vi "Autonomous Independent.vi"   [LabVIEW 2016]
doc: "This VI is called when autonomous begins, and will automatically be terminated when autonomous ends. You can carry out timed or sensor driven robot movement independently without needing to return to the caller."
uses:
  <vilib>/Rock Robotics/WPI/Relay/WPI_RelayValue.ctl
  <vilib>/Rock Robotics/WPI/Utilities/WPI_GetSetVariantRefNum.vi
  <vilib>/Rock Robotics/Network Tables/NT Read String.vi
  <vilib>/Rock Robotics/Network Tables/NT Read Number.vi
  <vilib>/Rock Robotics/Network Tables/NT Write Numeric Array.vi
panel:
  # "Be sure to right-click and choose Data Operations>>Make Current Value default if you want to save the array values with the VI"
types:
  T1 = typedef "WPI_JoystickDevRef.ctl" = cluster{"Device":T2}
  T2 = typedef "WPI_JoystickDeviceEnum.ctl" = enum16{"USB 0", "USB 1", "USB 2", "USB 3", "USB 4", "USB 5"}
  T3 = typedef "WPI_ServoDeviceRef.ctl" = cluster{"DeviceStatus":errorcluster, "PWM Channel":T4, "DeadBand":T5}
  T4 = typedef "FPGA_DIOPWMChannel.ctl" = enum8{"PWM 0", "PWM 1", "PWM 2", "PWM 3", "PWM 4", "PWM 5", "PWM 6", "PWM 7", "PWM 8", "PWM 9", "PWM MXP 0", "PWM MXP 1", "PWM MXP 2", "PWM MXP 3", "PWM MXP 4", "PWM MXP 5", "PWM MXP 6", "PWM MXP 7", "PWM MXP 8", "PWM MXP 9", "Invalid"}
  T5 = typedef "WPI_PWMDeadband.ctl" = cluster{"Name":string, "maxPositivePwm":i32, "minPositivePwm":i32, "centerPwm":i32, "maxNegativePwm":i32, "minNegativePwm":i32, "angularRange":u16}
  T6 = typedef "WPI_RelayValue.ctl" = enum16{"Off", "On", "Forward", "Reverse"}
  T7 = typedef "WPI_SwitchDevRef.ctl" = cluster{"DevStatus":errorcluster, "DIO Channel":T8, "CntIndex":T9, "Normally Closed":bool}
  T8 = typedef "FPGA_DIOChannel.ctl" = enum8{"DIO 0", "DIO 1", "DIO 2", "DIO 3", "DIO 4", "DIO 5", "DIO 6", "DIO 7", "DIO 8", "DIO 9", "DIO MXP 0", "DIO MXP 1", "DIO MXP 2", "DIO MXP 3", "DIO MXP 4", "DIO MXP 5", "DIO MXP 6", "DIO MXP 7", "DIO MXP 8", "DIO MXP 9", "DIO MXP 10", "DIO MXP 11", "DIO MXP 12", "DIO MXP 13", "DIO MXP 14", "DIO MXP 15", "SPI Port CS1", "SPI Port CS2", "SPI Port CS3", "SPI Port MISO", "SPI Port MOSI", "Invalid"}
  T9 = typedef "FPGA_CounterCtrSystemIndex.ctl" = enum8{"Ctr 0", "Ctr 1", "Ctr 2", "Ctr 3", "Ctr 4", "Ctr 5", "Ctr 6", "Ctr 7", "Invalid"}
  T10 = typedef "WPI_RelayDevRef.ctl" = cluster{"DevStatus":errorcluster, "Relay Channel":T11, "Relay Direction":T12}
  T11 = typedef "FPGA_DIORelayChannel.ctl" = enum8{"Relay 0", "Relay 1", "Relay 2", "Relay 3", "Invalid"}
  T12 = typedef "WPI_RelayDirection.ctl" = enum16{"Both directions", "Forward only", "Reverse only"}
  T13 = typedef "WPI_RobotDriveDevRef.ctl" = cluster{"DevStatus":errorcluster, "Motors[]":T14[], "Square Inputs":bool, "Max Output":dbl}
  T14 = typedef "WPI_MotorControlDeviceRef.ctl" = cluster{"DeviceStatus":errorcluster, "Type":T15, "PWM":cluster{"PWM Channel":T4, "DeadBand":T5}, "CAN":cluster{"Device Number":u8, "SetOutput VI Ref":variant, "GetOutput VI Ref":variant, "Enable VI Ref":variant, "Disable VI Ref":variant, "Data":variant}, "Invert":bool}
  T15 = typedef "WPI_MotorControlType.ctl" = enum16{"PWM", "CAN"}
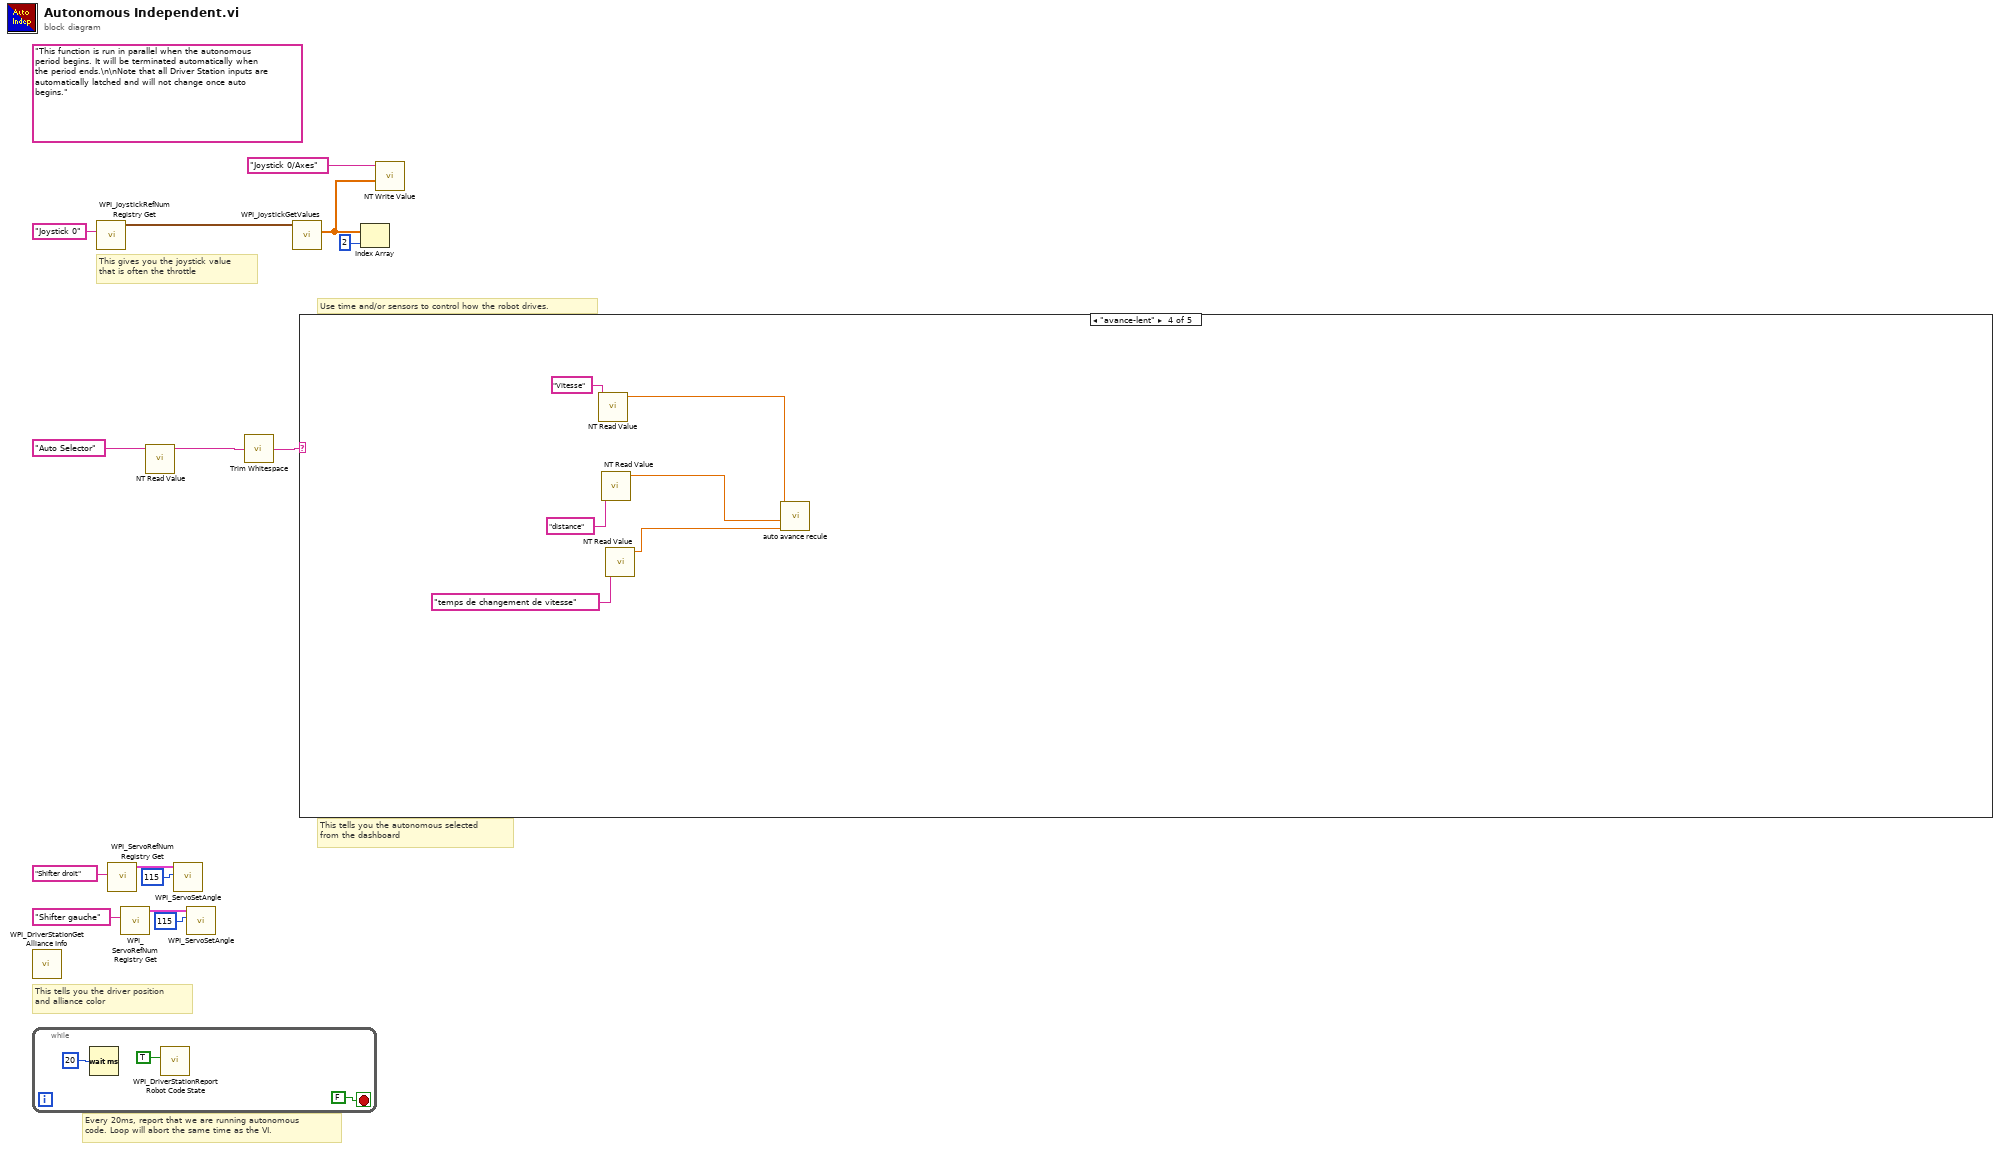
[diagram p0: block diagram]
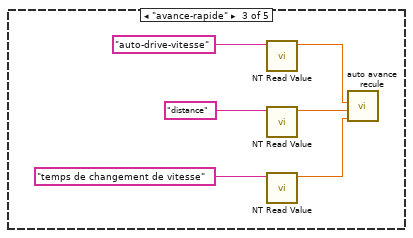
[diagram p4: hidden frame]
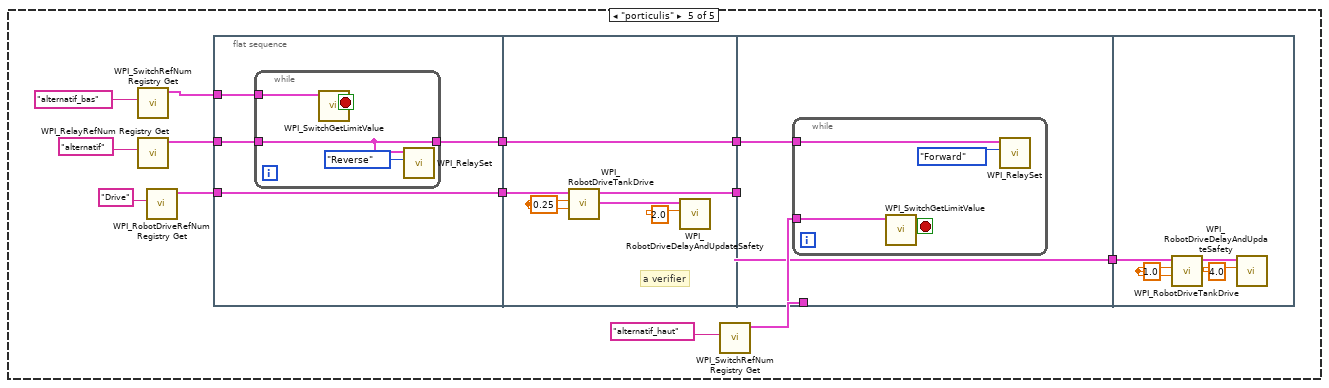
[diagram p5: hidden frame]
diagram:
  (unwired) "This function is run in parallel when the autonomous period begins. It will be terminated automatically when the period ends.\n\nNote that all Driver Station inputs are automatically latched and will not change once auto begins."
  # "This tells you the autonomous selected\nfrom the dashboard"
  # "Every 20ms, report that we are running autonomous\ncode. Loop will abort the same time as the VI."
  # "This gives you the joystick value\nthat is often the throttle"
  # "Use time and/or sensors to control how the robot drives."
  # "This tells you the driver position\nand alliance color"
  n1 = call <vilib>:"WPI_DriverStationGet Alliance Info.vi"() -> ()  [unwired: 12 out]
  n2 = while {
    stop <- FALSE stop-if-true
    n3 = Wait (ms)(milliseconds to wait=u32 20) -> ()  [unwired: 1 out]
    n4 = call <vilib>:"WPI_DriverStationReport Robot Code State.vi"("Autonomous"=TRUE) -> ()  [unwired: 10 in, 1 out]
  }
  n5 = call <vilib>:"WPI_JoystickRefNum Registry Get.vi"("refnum name"="Joystick 0") -> ("JoystickDevRef"=w13:T1)  [unwired: 1 in, 9 out]
  n6 = call <vilib>:"WPI_ServoRefNum Registry Get.vi"("refnum name"="Shifter droit") -> ("ServoDeviceRef"=w5:T3)  [unwired: 9 in, 1 out]
  n7 = call <vilib>:"WPI_ServoRefNum Registry Get.vi"("refnum name"="Shifter gauche") -> ("ServoDeviceRef"=w3:T3)  [unwired: 9 in, 1 out]
  n8 = call-poly <vilib>:"NT Read Value.vi"("Name"="Auto Selector") -> ("String"=w1:string)  [unwired: 9 in, 1 out]
  n9 = call <vilib>:"WPI_ServoSetAngle.vi"("Angle"=115, "ServoDeviceRef"=w5) -> ()  [unwired: 8 in, 2 out]
  n10 = call <vilib>:"WPI_ServoSetAngle.vi"("Angle"=115, "ServoDeviceRef"=w3) -> ()  [unwired: 8 in, 2 out]
  n11 = call <vilib>:"Trim Whitespace.vi"("string"=w1) -> ("trimmed string"=w2:string)  [unwired: 1 in]
  n12 = call <vilib>:"WPI_JoystickGetValues.vi"("JoystickDevRef"=w13) -> ("Axes"=w10:dbl[])  [unwired: 6 in, 4 out]
  n13 = case shown="\"avance-lent\"" w2 {
    frame Default {
      # "You can put your main auto here, or you can right-click on the case and make any\nother frame be the default case."
      # "This is the frame that will execute if no selection is made, or if it is not recognized"
    }
    frame "rien" {
    }
    frame "avance-rapide" {
      n14 = call-poly <vilib>:"NT Read Value.vi"("Name"="auto-drive-vitesse") -> ("Numeric"=w23:dbl)  [unwired: 9 in, 1 out]
      n15 = call-poly <vilib>:"NT Read Value.vi"("Name"="distance") -> ("Numeric"=w18:dbl)  [unwired: 9 in, 1 out]
      n16 = call-poly <vilib>:"NT Read Value.vi"("Name"="temps de changement de vitesse") -> ("Numeric"=w19:dbl)  [unwired: 9 in, 1 out]
      n17 = call "auto avance recule.vi"("temps de changement de direction"=w19, "temps"=w18, "vitesse"=w23) -> ()  [unwired: 9 in]
    }
    frame "avance-lent" {
      n18 = call-poly <vilib>:"NT Read Value.vi"("Name"="Vitesse") -> ("Numeric"=w29:dbl)  [unwired: 9 in, 1 out]
      n19 = call-poly <vilib>:"NT Read Value.vi"("Name"="distance") -> ("Numeric"=w24:dbl)  [unwired: 9 in, 1 out]
      n20 = call-poly <vilib>:"NT Read Value.vi"("Name"="temps de changement de vitesse") -> ("Numeric"=w25:dbl)  [unwired: 9 in, 1 out]
      n21 = call "auto avance recule.vi"("temps de changement de direction"=w25, "temps"=w24, "vitesse"=w29) -> ()  [unwired: 9 in]
    }
    frame "porticulis" {
      n22 = call <vilib>:"WPI_SwitchRefNum Registry Get.vi"("refnum name"="alternatif_bas") -> ("SwitchDevRef"=w36:T7)  [unwired: 9 in, 1 out]
      n23 = call <vilib>:"WPI_RelayRefNum Registry Get.vi"("refnum name"="alternatif") -> ("RelayDevRef"=w38:T10)  [unwired: 9 in, 1 out]
      n24 = call <vilib>:"WPI_RobotDriveRefNum Registry Get.vi"("refnum name"="Drive") -> ("RobotDriveDevRef"=w41:T13)  [unwired: 9 in, 1 out]
      n25 = flat-sequence {
        tunnel: w41 -> [w46]
        tunnel: [w46] -> w40
        tunnel: w38 -> [w45]
        tunnel: w36 -> [w44]
        tunnel: [w43] -> w33
        tunnel: w40 -> [w55]
        tunnel: w33 -> [w52]
        tunnel: [w52] -> w32
        tunnel: [w51] -> w31
        tunnel: w34 -> [w58]
        tunnel: w32 -> [w57]
        tunnel: w31 -> [w56]
        tunnel: [w56] -> w30
        tunnel: w30 -> [w63]
        frame #0 {
          n26 = while {
            tunnel: w45 -> [w47]
            tunnel: w44 -> [w49]
            tunnel: [w47] -> w43
            stop <- w48 stop-if-true
            n27 = call <vilib>:"WPI_SwitchGetLimitValue.vi"("SwitchDevRef"=w49) -> ("Switch Pressed"=w48:bool)  [unwired: 8 in, 2 out]
            n28 = call <vilib>:"WPI_RelaySet.vi"("RelayValue"=WPI_RelayValue."Reverse", "RelayDevRef"=w47) -> ()  [unwired: 8 in, 2 out]
          }
        }
        frame #1 {
          w54 = 0.25 ("Left axis value")
          # "a verifier"
          n29 = call <vilib>:"WPI_RobotDriveTankDrive.vi"("Right axis value"=w54, "Left axis value"=w54, "RobotDriveDevRef"=w55) -> ("RobotDriveDevRef"=w51:T13)  [unwired: 6 in, 2 out]
          n30 = call <vilib>:"WPI_RobotDriveDelayAndUpdateSafety.vi"("Delay (s)"=2.0, "RobotDriveDevRef"=w51) -> ()  [unwired: 8 in, 2 out]
        }
        frame #2 {
          n31 = while {
            tunnel: w57 -> [w61]
            tunnel: w58 -> [w60]
            stop <- w59 stop-if-true
            n32 = call <vilib>:"WPI_SwitchGetLimitValue.vi"("SwitchDevRef"=w60) -> ("Switch Pressed"=w59:bool)  [unwired: 8 in, 2 out]
            n33 = call <vilib>:"WPI_RelaySet.vi"("RelayValue"=WPI_RelayValue."Forward", "RelayDevRef"=w61) -> ()  [unwired: 8 in, 2 out]
          }
        }
        frame #3 {
          w65 = 1.0 ("Left axis value")
          n34 = call <vilib>:"WPI_RobotDriveTankDrive.vi"("Right axis value"=w65, "Left axis value"=w65, "RobotDriveDevRef"=w63) -> ("RobotDriveDevRef"=w66:T13)  [unwired: 6 in, 2 out]
          n35 = call <vilib>:"WPI_RobotDriveDelayAndUpdateSafety.vi"("Delay (s)"=4.0, "RobotDriveDevRef"=w66) -> ()  [unwired: 8 in, 2 out]
        }
      }
      n36 = call <vilib>:"WPI_SwitchRefNum Registry Get.vi"("refnum name"="alternatif_haut") -> ("SwitchDevRef"=w34:T7)  [unwired: 9 in, 1 out]
    }
  }
  n37 = Index Array(array=w10, index=2) -> ()  [unwired: 1 out]
  n38 = call-poly <vilib>:"NT Write Value.vi"("Numeric Array"=w10, "Name"="Joystick 0/Axes") -> ()  [unwired: 9 in, 1 out]
